vi "CfgManager Main Test Suite.vi"() -> ()   [LabVIEW 2013]
uses:
  source/Cache/ConfigManager.Cache.lvclass
  <vilib>/addons/_JKI Toolkits/Caraya/classes/Assert/Assert True.vi
  source/Manager/Write.vi
  source/Manager/ConfigManager.lvclass
  <vilib>/addons/_JKI Toolkits/Caraya/classes/Test/Test.lvclass
  <vilib>/addons/_JKI Toolkits/Caraya/classes/Assert/Assert.lvclass
panel:
  out "Values":variant[](array[variant])
  out "Keys":string[](array[string])
  out "Keys":string[](array[string])
  out "error out":errorcluster
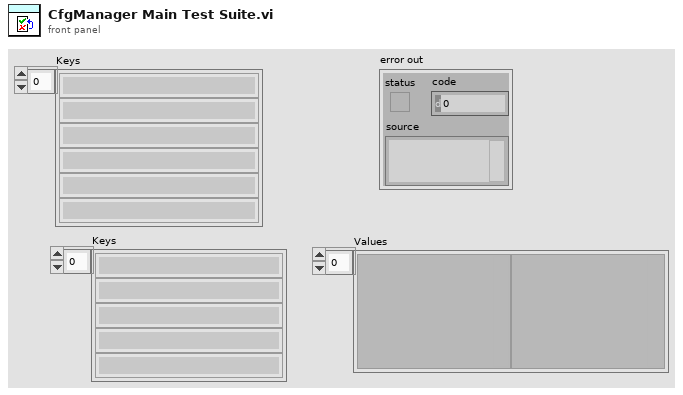
[diagram p1: front panel]
types:
  T1 = cluster{"P":dbl, "Type":enum16{"Manual", "Automatic"}}
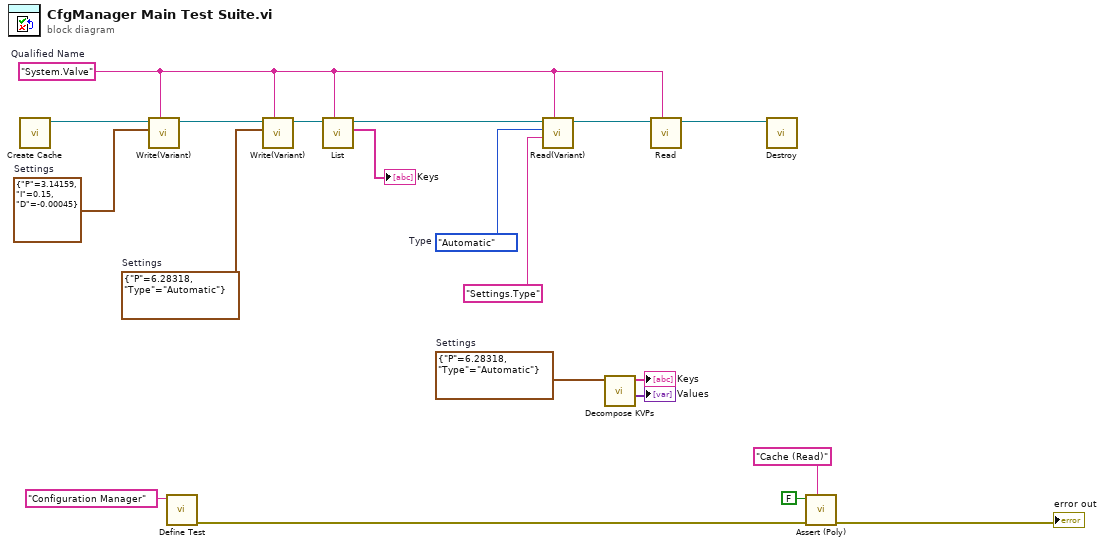
[diagram p0: block diagram]
diagram:
  w3 = T1 {"P"=6.28318, "Type"=enum."Automatic"}  # Settings
  w5 = enum16{"Manual", "Automatic"}."Automatic"  # Type
  w10 = T1 {"P"=6.28318, "Type"=enum."Automatic"}  # Settings
  w20 = cluster{"P":dbl, "I":dbl, "D":dbl} {"P"=3.14159, "I"=0.15, "D"=-0.00045}  # Settings
  w6 = "System.Valve"  # Qualified Name
  n1 = call "Create Cache.vi"() -> ("ConfigManager.Cache"=w19:refnum<class "ConfigManager.Cache.lvclass">)  [unwired: 11 in]
  n2 = call "Write(Variant).vi"("Qualified Name"=w6, "value"=w20, "ConfigManager in"=w19) -> ("ConfigManager out"=w12:refnum<class "ConfigManager.Cache.lvclass">)  [unwired: 6 in, 2 out]
  n3 = call <vilib>:"Define Test.vi"("Label (VI Title)"="Configuration Manager") -> ("error out"=w17:errorcluster)  [unwired: 10 in]
  n4 = call "Write(Variant).vi"("Qualified Name"=w6, "value"=w10, "ConfigManager in"=w12) -> ("ConfigManager out"=w11:refnum<class "ConfigManager.Cache.lvclass">)  [unwired: 6 in, 2 out]
  n5 = call "List.vi"("Qualified Name"=w6, "ConfigManager in"=w11) -> ("Keys"=→"Keys":string[], "ConfigManager out"=w9:refnum<class "ConfigManager.Cache.lvclass">)  [unwired: 7 in, 1 out]
  n6 = call "Read(Variant).vi"("Qualified Name"=w6, "Name (empty: type name)"="Settings.Type", "Type"=w5, "ConfigManager in"=w9) -> ("ConfigManager out"=w8:refnum<class "ConfigManager.Cache.lvclass">)  [unwired: 3 in, 4 out]
  n7 = call "Decompose KVPs.vi"("value"=w3) -> ("Values"=→"Values":variant[], "Keys"=→"Keys":string[])  [unwired: 9 in]
  n8 = call "Read.vi"("Qualified Name"=w6, "ConfigManager in"=w8) -> ("ConfigManager out"=w7:refnum<class "ConfigManager.Cache.lvclass">)  [unwired: 4 in, 5 out]
  n9 = call-dynamic "Destroy.vi"("ConfigManager.Cache in"=w7) -> ()  [unwired: 9 in, 2 out]
  n10 = call-poly <vilib>:"Assert (Poly).vi"("Label"="Cache (Read)", "error in (no error)"=w17, "True?"=FALSE) -> ("error out"=→"error out":errorcluster)  [unwired: 8 in]
